vi "Write Header to Error Log File.vi"(8 "error in (no error)":errorcluster, 11 "Text Log In":refnum<class "Text Log.lvclass">) -> (0 "error out":errorcluster, 3 "Text Log Out":refnum<class "Text Log.lvclass">)   [LabVIEW 2020, in "Error Log Classes.lvlib" / "Text Log.lvclass"]
uses:
  Text Log.lvclass
  Text Log.lvclass/Text Log.ctl
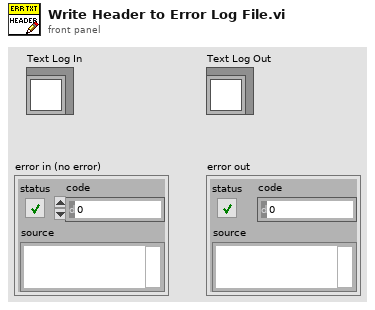
[diagram p1: front panel]
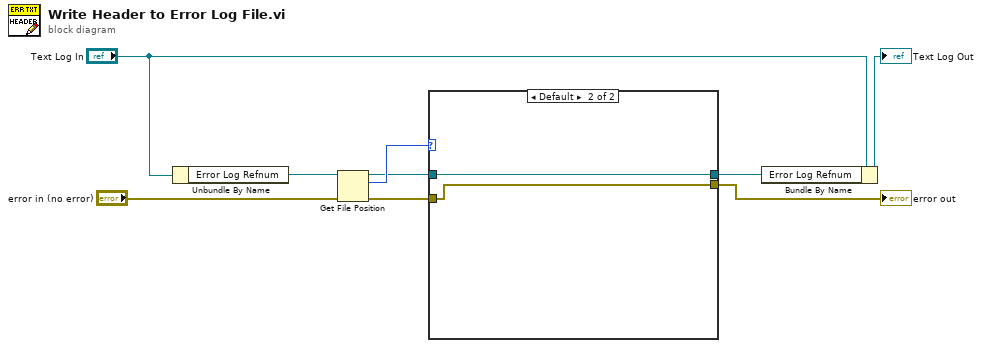
[diagram p0: block diagram]
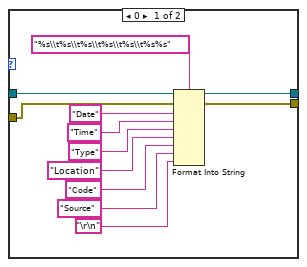
[diagram p2: hidden frame]
diagram:
  n1 = Unbundle By Name("Text Log In") -> ("Error Log Refnum"=w7:refnum<file>)
  n2 = Get File Position(4:"error in (no error)", 7:w7) -> (0:w3:errorcluster, 2:w5:i64, 3:w4:refnum<file>)
  n3 = case shown="Default" w5 {
    tunnel: w4 -> [w20 w23]
    tunnel: [w19 w23] -> w6
    tunnel: w3 -> [w11 w22]
    tunnel: [w10 w22] -> w8
    frame 0 {
      n4 = Format Into String(format string="%s\\t%s\\t%s\\t%s\\t%s\\t%s%s", initial string=w20, error in=w11, "Date" ("input 1"), "Time" ("input 1"), "Type" ("input 1"), "Location" ("input 1"), "Code" ("input 1"), "Source" ("input 1"), "\r\n") -> (resulting string=w19:refnum<file>, error out=w10:errorcluster)
    }
    frame Default {
    }
  }
  "error out" <- w8
  n5 = Bundle By Name(cluster="Text Log In", "Error Log Refnum"=w6) -> (→"Text Log Out":refnum<class "Text Log.lvclass">)
